vi "Check if password valid -active -expired.vi"(7 "Warning days":i32=30, 9 "Password":string, 10 "User access cluster":T1 {"Expire sec" format="%.2f"}, 11 "Expiration enabled?":bool) -> (1 "Valid & current?":bool, 2 "Expired?":bool, 3 "Active?":bool)   [LabVIEW 2012]
doc: "First checks to see if active? =F or expired? = T (if \"Expiration enabled?\" =T) in the user access cluster. If so, the remaining steps are skipped and this vi returns corresponding states for \"Active?' and \"Expired?\" and \"Valid and current?' = F.\n\nOtherwise, this vi then checks to see if password matches the password in the user access cluster. (Case insensitive). If not, vi returns \"Valid & current?\" = F.\n\nIf the pasword does match and \"Expiration enabled?\" =T, this vi then compares the current epoch seconds with the 'expire sec\" in the user access cluster. If current sec is greater than this vi returns \"Valid & current?\" = F. If the current secs is less than this value it returns \"Valid & current?\" = T.\n\nIf the days remaining to expiration of the password is less than \"warning days\" and \"Expiration enabled?\" =T the user is given a pop-up warning. All other warnings and notifications to the user are handled by higher level vis."
uses:
  User Access Type defs/User access cluster.ctl
  User Access Type defs/Security level U8.ctl
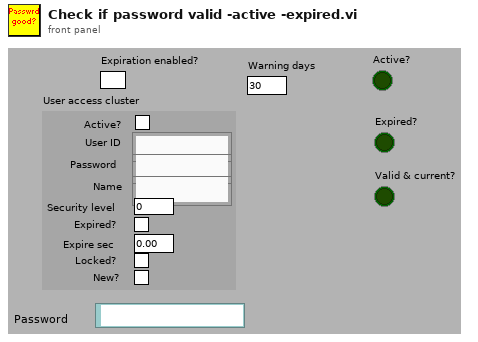
[diagram p1: front panel]
types:
  T1 = typedef "User access cluster.ctl" = cluster{"Active?":bool, "User ID":string, "Password":string, "Name":string, "Security level":T2, "Expired?":bool, "Expire sec":dbl, "Locked?":bool, "New?":bool}
  T2 = typedef "Security level U8.ctl" = u8
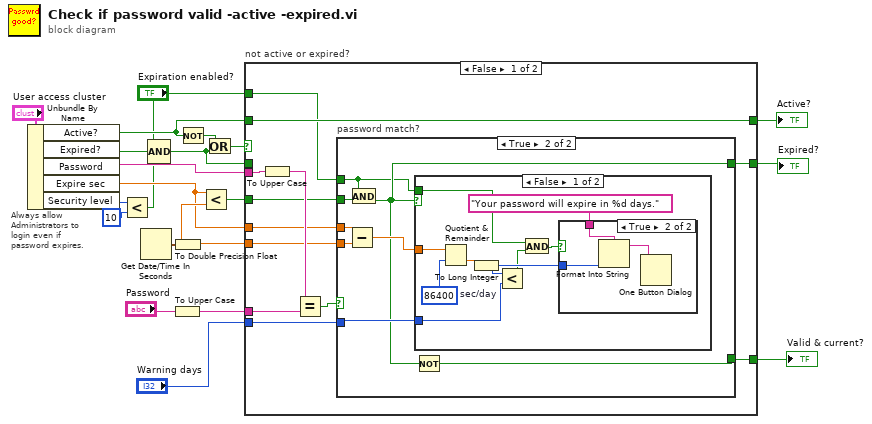
[diagram p0: block diagram]
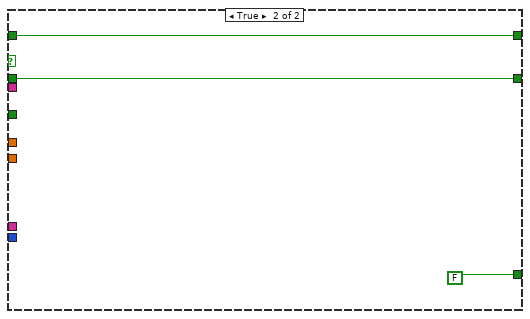
[diagram p5: hidden frame]
diagram:
  # "Always allow Administrators to login even if password expires."
  n1 = Unbundle By Name("User access cluster") -> ("Active?"=w14:bool, "Expired?"=w7:bool, "Password"=w20:string, "Expire sec"=w9:dbl, "Security level"=w4:T2)
  n2 = Less?(x=w4, y=T2 10) -> (x < y?=w2:bool)
  n3 = Get Date/Time In Seconds() -> (seconds since 1Jan1904=w1:timestamp)
  n4 = Compound Arithmetic op=AND("Expiration enabled?", w7, w2) -> (w5:bool)
  n5 = To Upper Case(1:"Password") -> (0:w19:string)
  n6 = To Double Precision Float(number=w1) -> (double precision float=w10:dbl)
  n7 = Not(x=w14) -> (.not. x?=w21:bool)
  n8 = Less?(x=w9, y=w10) -> (x < y?=w11:bool)
  n9 = Or(x=w21, y=w5) -> (x .or. y?=w16:bool)
  n10 = case "not active or expired?" shown="False" w16 {
    tunnel: w20 -> [w33 _]
    tunnel: w19 -> [w31 _]
    tunnel: [w28 FALSE ("Valid & current?")] -> w15
    tunnel: [w30 w56] -> w13
    tunnel: w14 -> [w30 w56]
    tunnel: [w27 w55] -> w12
    tunnel: w5 -> [_ w55]
    tunnel: w11 -> [w26 _]
    tunnel: w10 -> [w25 _]
    tunnel: w9 -> [w24 _]
    tunnel: "Warning days" -> [w23 _]
    tunnel: "Expiration enabled?" -> [w22 _]
    frame False {
      n11 = To Upper Case(1:w33) -> (0:w32:string)
      n12 = Equal?(x=w32, y=w31) -> (x = y?=w29:bool)
      n13 = case "password match?" shown="True" w29 {
        selector: w29 -> [w34 _]
        tunnel: [w34 w42] -> w28
        tunnel: [w34 w36] -> w27
        tunnel: w26 -> [_ w37]
        tunnel: w25 -> [_ w38]
        tunnel: w24 -> [_ w39]
        tunnel: w23 -> [_ w41]
        tunnel: w22 -> [_ w35]
        frame False {
        }
        frame True {
          n14 = Subtract(x=w39, y=w38) -> (x-y=w40:dbl)
          n15 = And(x=w35, y=w37) -> (x .and. y?=w36:bool)
          n16 = Not(x=w36) -> (.not. x?=w42:bool)
          n17 = case shown="False" w36 {
            tunnel: w41 -> [w51 _]
            tunnel: w40 -> [w50 _]
            tunnel: w35 -> [w45 _]
            frame False {
              w49 = 86400  # sec/day
              n18 = Quotient & Remainder(x=w50, y=w49) -> (floor(x/y)=w48:dbl)  [unwired: 1 out]
              n19 = To Long Integer(number=w48) -> (32bit integer=w47:i32)
              n20 = Less?(x=w47, y=w51) -> (x < y?=w44:bool)
              n21 = And(x=w45, y=w44) -> (x .and. y?=w43:bool)
              n22 = case shown="True" w43 {
                tunnel: w47 -> [_ w54]
                tunnel: "Your password will expire in %d days." ("format string") -> [_ w53]
                frame False {
                }
                frame True {
                  n23 = Format Into String(format string=w53, w54) -> (resulting string=w52:string)  [unwired: 2 in, 1 out]
                  n24 = One Button Dialog(message=w52) -> ()  [unwired: 2 out]
                }
              }
            }
            frame True {
            }
          }
        }
      }
    }
    frame True {
    }
  }
  "Active?" <- w13
  "Expired?" <- w12
  "Valid & current?" <- w15
